vi "Utility Greeter.vi"(9 "Name":string, 10 "Greeting":string) -> (2 "Output":string)   [LabVIEW 2026]
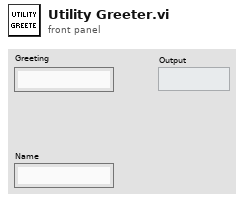
[diagram p1: front panel]
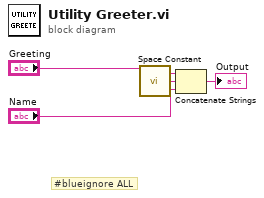
[diagram p0: block diagram]
diagram:
  # "#blueignore ALL"
  n1 = call <vilib>:"Space Constant.vi"() -> ("String"=w2:string)
  n2 = Concatenate Strings("Greeting", w2, "Name") -> (→"Output":string)
